vi "Create lvlib Folder.vi"(8 "Template Library Name":string, 9 "Template Name":string, 10 "Project:Active Project":refnum<vi>) -> (1 "Library Path":path, 2 "Library Folder Path":path)   [LabVIEW 2021, in "_Template.lvlib" / "Script.lvlib" / "Script.lvclass"]
uses:
  Script/Script.lvclass
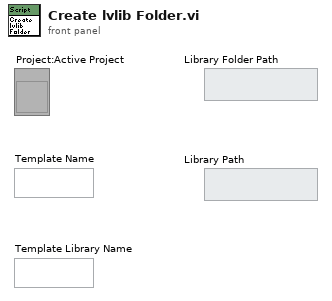
[diagram p1: front panel]
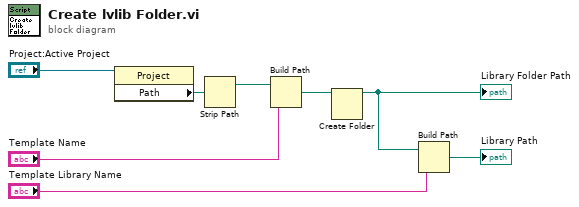
[diagram p0: block diagram]
diagram:
  n1 = property class="Project"(reference="Project:Active Project") -> ("Path"=w6:path)  [unwired: 1 in, 2 out]
  n2 = Strip Path(path=w6) -> (stripped path=w7:path)  [unwired: 1 out]
  n3 = Build Path(base path=w7, name or relative path="Template Name") -> (appended path=w8:path)
  n4 = Create Folder(path (use dialog)=w8) -> (created path=w4:path)  [unwired: 2 in, 2 out]
  "Library Folder Path" <- w4
  n5 = Build Path(base path=w4, name or relative path="Template Library Name") -> (appended path=→"Library Path":path)
